vi "Init Buffers.vi"(8 "error in (no error)":errorcluster, 11 "Terminal in":refnum<class "Terminal.lvclass">) -> (0 "error out":errorcluster, 3 "Terminal out":refnum<class "Terminal.lvclass">)   [LabVIEW 2020, in "Terminal.lvlib" / "Terminal.lvclass"]
uses:
  Terminal.lvclass
  Terminal.lvclass/Terminal.ctl
  TermBuffer/TermBuffer.lvclass
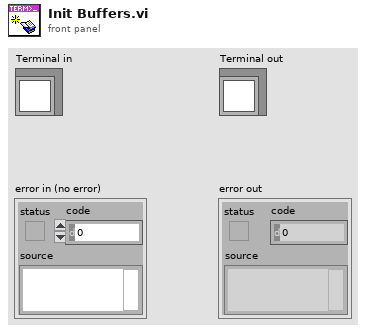
[diagram p1: front panel]
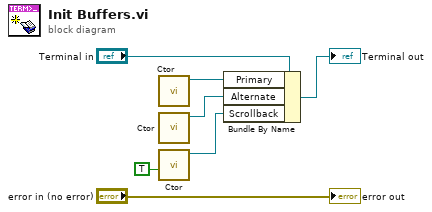
[diagram p0: block diagram]
diagram:
  n1 = call "Ctor.vi"() -> ("TermBuffer out"=w3:refnum<class "TermBuffer.lvclass">)  [unwired: 10 in, 1 out]
  n2 = call "Ctor.vi"() -> ("TermBuffer out"=w1:refnum<class "TermBuffer.lvclass">)  [unwired: 10 in, 1 out]
  n3 = call "Ctor.vi"("Is Scrollback? (F)"=TRUE) -> ("TermBuffer out"=w2:refnum<class "TermBuffer.lvclass">)  [unwired: 9 in, 1 out]
  n4 = Bundle By Name(cluster="Terminal in", "Primary"=w3, "Alternate"=w1, "Scrollback"=w2) -> (→"Terminal out":refnum<class "Terminal.lvclass">)
  "error out" <- "error in (no error)"
